vi "getDisabledRows.vi"(8 "error in (no error)":errorcluster, 11 "CategoryList in":refnum<class "CategoryList.lvclass">) -> (0 "error out":errorcluster, 2 "Highlighted Rows":i32[](array[numeric]), 3 "CategoryList out":refnum<class "CategoryList.lvclass">)   [LabVIEW 2020, in "CategoryList.lvclass"]
uses:
  CategoryList.lvclass
  CategoryList.lvclass/CategoryList.ctl
  Category/Category.lvclass
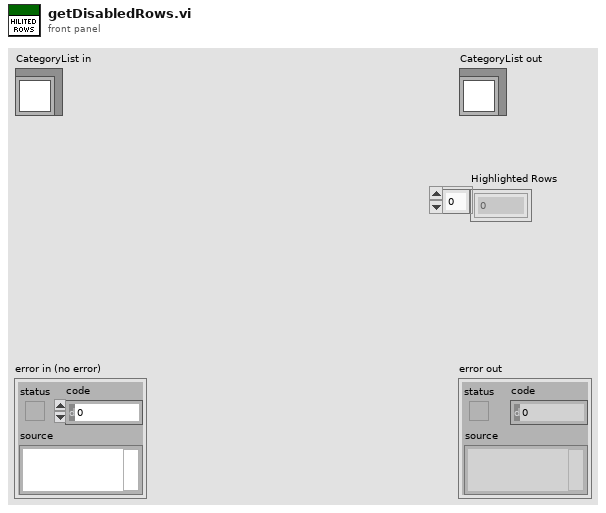
[diagram p1: front panel]
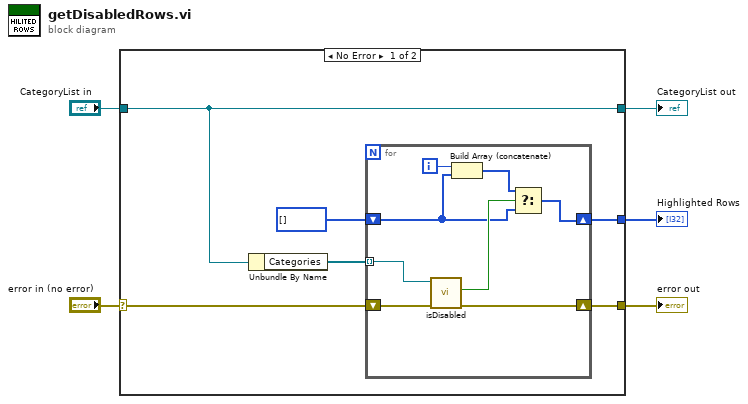
[diagram p0: block diagram]
diagram:
  n1 = case shown="No Error" "error in (no error)" {
    selector: "error in (no error)" -> [w9 w21]
    tunnel: [w8 w21] -> w4
    tunnel: [w11 w20] -> w2
    tunnel: "CategoryList in" -> [w11 w20]
    tunnel: [w6 _] -> w1
    frame No Error {
      n2 = Unbundle By Name(w11) -> ("Categories"=w10:refnum<class "Category.lvclass">[])
      n3 = for {
        tunnel: w10 -> [w18] mode=indexing
        shift-right: [w17] -> w8
        shift-left: w9 -> [w19]
        shift-right: [w15] -> w6
        shift-left: i32[] [] ("Highlighted Rows") -> [w13]
        i -> [w14]
        n4 = call-dynamic "isDisabled.vi"("error in (no error)"=w19, "Category in"=w18) -> ("error out"=w17:errorcluster, "Disabled?"=w16:bool)  [unwired: 7 in, 1 out]
        n5 = Build Array (concatenate)(w14, w13) -> (w12:i32[])
        n6 = Select(t=w12, s=w16, f=w13) -> (s? t:f=w15:i32[])
      }
    }
    frame Error {
    }
  }
  "error out" <- w4
  "CategoryList out" <- w2
  "Highlighted Rows" <- w1
